vi "Trip Log and Trip Monitor.vi"(8 "error in (no error)":errorcluster, 11 "main ref":T1) -> (0 "error out":errorcluster)   [LabVIEW 2025]
uses:
  controls/LAB-IQ UI Data.ctl
  <vilib>/Utility/error.llb/Trim Whitespace One-Sided.vi
panel:
  in  "millisecond multiple":u32=5
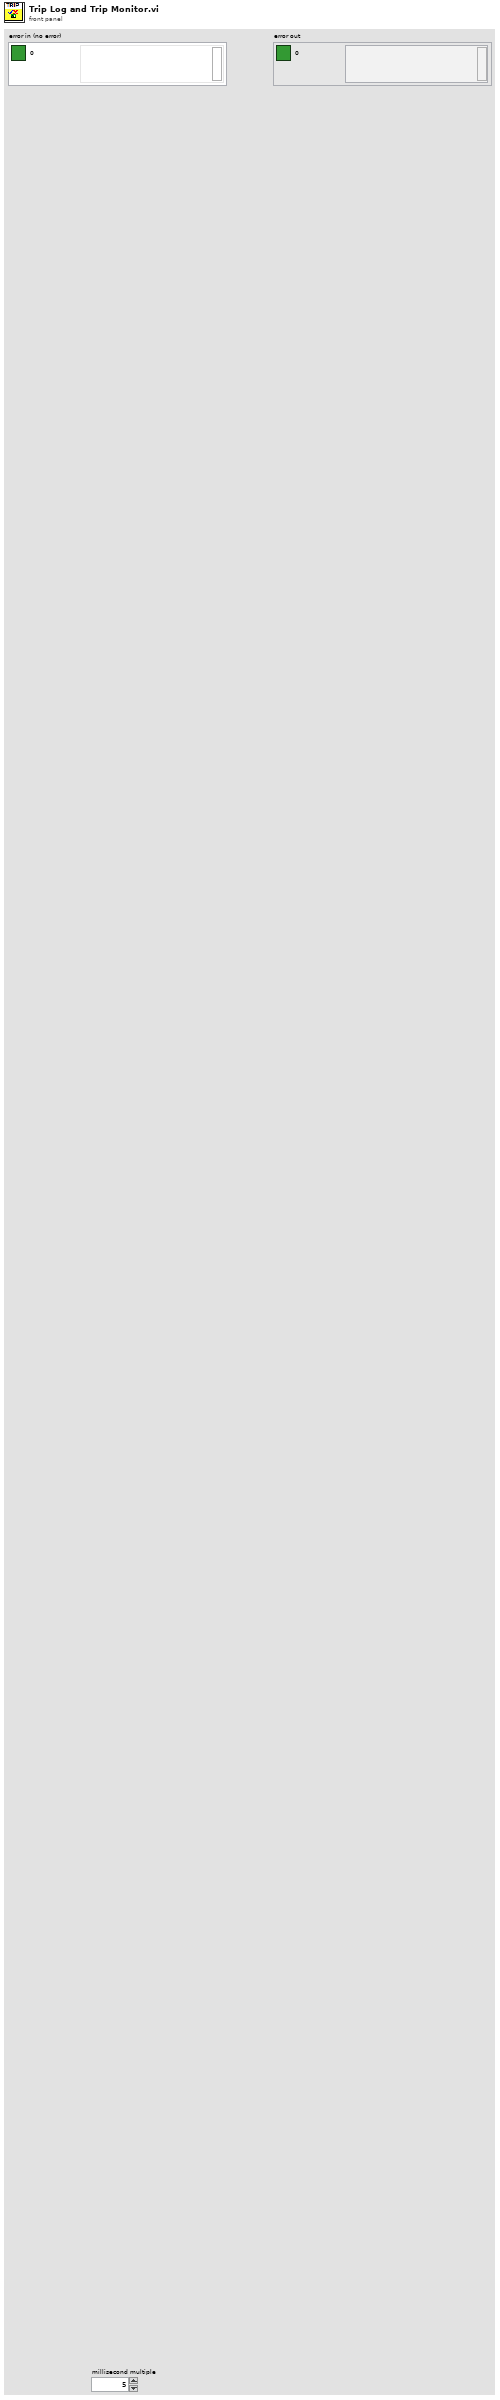
[diagram p1: front panel]
types:
  T1 = typedef "LAB-IQ UI Data.ctl" = cluster{"Main Home Screen":cluster{"GUI":refnum<vi>, "Platform Settings":refnum<vi>, "Configure":refnum<vi>, "Home":refnum<vi>, "EXIT":refnum<vi>, "service 2":refnum<vi>, "MainPage":refnum<vi>, "Analysis":refnum<vi>}, "Platform Settings":cluster{"mm/s  Surge":refnum<vi>, "Update Surge Speed":refnum<vi>, "Drive Error":refnum<vi>, "Disable Axis Jog Soft Limits":refnum<vi>, "mm/s  Sway":refnum<vi>, "Sway and Surge COM Status":refnum<vi>, "Heave COM Status":refnum<vi>, "Enable Platform":refnum<vi>, "Surge Forward Main":refnum<vi>, "Sway Right Main":refnum<vi>, "Sway Left Main":refnum<vi>, "Heave Down Main":refnum<vi>, "Heave Up main":refnum<vi>, "Update Sway Speed":refnum<vi>, "Update Heave Speed":refnum<vi>, "mm/s Heave":refnum<vi>, "mm/sec":refnum<vi>, "mm":refnum<vi>, "Surge Backward Main":refnum<vi>}, "Analysis Screen":cluster{"Analysis Home":refnum<vi>, "Surface Analysis":refnum<vi>, "Imaging":refnum<vi>, "Image Analysis":refnum<vi>, "Post Analysis":refnum<vi>}, "Config Screen":cluster{"Select Load Head":refnum<vi>, "Notes :":refnum<vi>, "FILE":refnum<vi>, "Sample ID :":refnum<vi>, "Operator ID :":refnum<vi>, "Operator Name :":refnum<vi>, "Auto":refnum<vi>}, "Motion Module":cluster{"zNL":refnum<vi>, "NL disp":refnum<vi>, "Rotary Tab":refnum<vi>, "Motion Direction:  3":refnum<vi>, "E.Velocity 2":refnum<vi>, "e.v/ssr 2":refnum<vi>, "Enter Fixed E.Velocity 2":refnum<vi>, "Enter Final SRR 2":refnum<vi>, "Enter initial SRR 2":refnum<vi>, "Enter Fixed SRR 2":refnum<vi>, "Enter the Final E.Velocity (m/s) 2":refnum<vi>, "Enter initial E.Velocity (m/s) 2":refnum<vi>, "Final Speed (RPM) 3":refnum<vi>, "Initial Speed (RPM) 2":refnum<vi>, "Enter the Final Velocity (m/s) 3":refnum<vi>, "Enter initial Velocity (m/s)  3":refnum<vi>, "Ramp Up 2":refnum<vi>, "TEST SELECTION":refnum<vi>, "SPEED SELECTION : ":refnum<vi>, "Angular Oscillation Set":refnum<vi>, "Traction":refnum<vi>, "Step Speed":refnum<vi>, "StepTable For Load-Speed":refnum<vi>, "StepTable For Speed":refnum<vi>, "Surge Forward MM":refnum<vi>, "Surge Backward MM":refnum<vi>, "M3 Image":refnum<vi>, "String 39":refnum<vi>, "Sway Left MM":refnum<vi>, "Sway Right MM":refnum<vi>, "Disable Axis Jog Soft Limits":refnum<vi>, "mm":refnum<vi>, "Heave Down MM":refnum<vi>, "Heave Up MM":refnum<vi>, "Wear Track Diameter (mm)":refnum<vi>, "Set WTD":refnum<vi>, "HomeScratch":refnum<vi>, "HomeRot":refnum<vi>, "PlaceModule":refnum<vi>, "Enter the Angle (Deg)":refnum<vi>, "Enter the Frequency (Hz)":refnum<vi>, "Motion Mode:":refnum<vi>, "LR Sway":refnum<vi>, "Rot Hor":refnum<vi>, "Scratch":refnum<vi>, "LR Cam":refnum<vi>, "MMBack":refnum<vi>, "MMNext":refnum<vi>, "Rot Ver":refnum<vi>, "Rotary Module Selection":refnum<vi>, "calculate rotary":refnum<vi>, "SPEED SELECTION : rotary":refnum<vi>, "Import 2":refnum<vi>, "Save 2":refnum<vi>, "File Path :  2":refnum<vi>, "String 45":refnum<vi>, "StepTable For Speed 3":refnum<vi>, "Enter the Speed(mm/sec)":refnum<vi>, "Enter the Speed(RPM)":refnum<vi>, "Enter Scratch Speed (mm/s):":refnum<vi>, "SwaySpeed Set":refnum<vi>, "Scartch Offset":refnum<vi>, "Motion type:":refnum<vi>, "HomeScratch 2":refnum<vi>, "Enter Scratch length (mm):":refnum<vi>, "Wear Track Diameter":refnum<vi>, "Rotary Speed Exced":refnum<vi>, "Scratch Mode":refnum<vi>, "No of Scratch":refnum<vi>}, "Environmental control":cluster{"Humidity  Status  3":refnum<vi>, "Low Temp  Status  2":refnum<vi>, "TK4 status 2":refnum<vi>, "Stage Temperature":refnum<vi>, "Sample Temperature":refnum<vi>, "Humidity (Amb)":refnum<vi>, "Clear List":refnum<vi>, "Add to list":refnum<vi>, "Wear":refnum<vi>, "Vibration":refnum<vi>, "Humidity (Chamber)":refnum<vi>, "Temperature (Chamber)":refnum<vi>, "ECR ":refnum<vi>, "Temperature (Amb)":refnum<vi>, "Microphone":refnum<vi>, "Acoustic Emission 3":refnum<vi>, "SNext":refnum<vi>, "APBack":refnum<vi>, "Enter the Temperature (°C):":refnum<vi>, "Enter the Stage \nTemperature (°C):":refnum<vi>, "Enter the Humidity (%Rh):":refnum<vi>, "Low Temp":refnum<vi>, "High Temp":refnum<vi>, "Humidity":refnum<vi>, "Sensors Picked":refnum<vi>}, "About Screen":cluster{"Password":refnum<vi>, "Home Service":refnum<vi>, "Advanced Setting":refnum<vi>, "About Tab":refnum<vi>, "ECR Port:":refnum<vi>, "Ramp Port:":refnum<vi>, "Installation/Replacement completed":refnum<vi>, "Loahead":refnum<vi>, "Heave and Surge COM Port:":refnum<vi>, "Sway COM Port:":refnum<vi>, "Temp Modbus:":refnum<vi>, "Humidity Port:":refnum<vi>, "Edit Gain Constants":refnum<vi>, "Save Gain Constants":refnum<vi>}, "Main Screen":cluster{"Main Screen Tab":refnum<vi>, "Angle and Frequency":refnum<vi>, "Stroke (mm)":refnum<vi>, "Angle (Deg)":refnum<vi>, "Main Speed Tab":refnum<vi>, "MTM MOTOR DISPLAY":refnum<vi>, "Disc Speed (m/sec)":refnum<vi>, "Ball Speed (m/sec)":refnum<vi>, "Disc Speed (RPM)":refnum<vi>, "Ball Speed (RPM)":refnum<vi>, "SPEED TAB":refnum<vi>, "Speed (m/sec)":refnum<vi>, "Set Speed (m/sec)":refnum<vi>, "Speed (RPM)":refnum<vi>, "Set Speed":refnum<vi>, "Time Tab":refnum<vi>, "Time ( HH:MM:SS ) 2":refnum<vi>, "Test Duration":refnum<vi>, "Test Duration 4":refnum<vi>, "TEST CYCLE":refnum<vi>, "TOTAL CYCLES":refnum<vi>, "Set Load (N)":refnum<vi>, "Temp Tabs":refnum<vi>, "Heater":refnum<vi>, "TK4 status":refnum<vi>, "ChamberTemp":refnum<vi>, "SetTmp":refnum<vi>, "Controller  Status":refnum<vi>, "ChamberTemp 2":refnum<vi>, "SetTmp 2":refnum<vi>, "Controller  Status 2":refnum<vi>, "ChamberTemp 3":refnum<vi>, "SetTmp 3":refnum<vi>, "Cooling":refnum<vi>, "Load Communication":refnum<vi>, "Ambient \nTemperature":refnum<vi>, "HumCOMStatus":refnum<vi>, "Ambient\n Humidity":refnum<vi>, "Freq (Hz)":refnum<vi>, "Load En":refnum<vi>, "NLt":refnum<vi>, "zNL 2":refnum<vi>, "Humidity On":refnum<vi>, "humidity disp":refnum<vi>, "Set Humidity":refnum<vi>, "NL disp 2":refnum<vi>, "Humidity On 2":refnum<vi>, "humidity disp 2":refnum<vi>, "Set Humidity 2":refnum<vi>, "NL disp 3":refnum<vi>, "AppLoadSeq scratch":refnum<vi>, "Stop Scratch":refnum<vi>, "ClrLog":refnum<vi>, "Trip Log":refnum<vi>, "STOP":refnum<vi>, "Start Test":refnum<vi>, "Test status":refnum<vi>, "AR Led":refnum<vi>, "Data":refnum<vi>, "Health":refnum<vi>, "Sway COM Status":refnum<vi>, "Heave COM Status":refnum<vi>, "Grp Tab":refnum<vi>, "Sub Graph":refnum<vi>, "SD (mm)":refnum<vi>, "Siliding distance Reset Graph":refnum<vi>, "SDGp":refnum<vi>, "Humidity Reset Graph":refnum<vi>, "HumrGp":refnum<vi>, "Acoustic Emission (mV)":refnum<vi>, "Aqucostic Reset Graph":refnum<vi>, "gACQUOS":refnum<vi>, "ECR RESET":refnum<vi>, "ECR":refnum<vi>, "Temperature Reset":refnum<vi>, "Acoustic Emission (mV) 2":refnum<vi>, "Aqucostic Reset Graph 2":refnum<vi>, "gACQUOS 2":refnum<vi>, "ECR RESET 2":refnum<vi>, "ECR 2":refnum<vi>, "Temperature Reset 2":refnum<vi>, "Temperature (deg c)":refnum<vi>, "Speed Reset Graph":refnum<vi>, "Speed Tab":refnum<vi>, "MTM DISC  SPEED":refnum<vi>, "MTM BALL SPEED":refnum<vi>, "speed mm/sec":refnum<vi>, "Hymidity":refnum<vi>, "Humidity Disable trip":refnum<vi>, "CoF Trip  2":refnum<vi>, "Depth Trip":refnum<vi>, "Weart Deapth":refnum<vi>, "Depth Reset Graph":refnum<vi>, "Weart":refnum<vi>, "Depthz":refnum<vi>, "Depth (µm)":refnum<vi>, "WearGp":refnum<vi>, "NL Trip 2":refnum<vi>, "Load pid":refnum<vi>, "Load Disable Trip":refnum<vi>, "Load Reset Graph":refnum<vi>, "NL Display 4":refnum<vi>, "Main Chart 3":refnum<vi>, "BACK":refnum<vi>, "Depth Trip 2":refnum<vi>, "COF TRIP ":refnum<vi>, "Friction Force (N)":refnum<vi>, "FF Reset Graph":refnum<vi>, "FF Disable Trip":refnum<vi>, "FF TRIP":refnum<vi>, "COF Disable Trip":refnum<vi>, "COF Reset Graph":refnum<vi>, "Start Test Temp":refnum<vi>, "zFF":refnum<vi>, "Friction Force (N) Graph":refnum<vi>, "Coefficient of Friction":refnum<vi>, "Scratch Start Test":refnum<vi>, "FF Tab":refnum<vi>, "Cyclic Friction Force (N)":refnum<vi>, "CZ FF":refnum<vi>, "Cyclic Friction Force (N) Graph":refnum<vi>, "Cyclic Coefficient of Friction":refnum<vi>, "Cyclic FF TRIP":refnum<vi>, "Cyclic FF Disable Trip":refnum<vi>, "cyclic COF Disable Trip":refnum<vi>, "cyclic COF TRIP":refnum<vi>, "cyclic COF Reset Graph":refnum<vi>, "Cyclic FF Reset Graph":refnum<vi>, "Test Trip":refnum<vi>, "Multi Scratch Pass":refnum<vi>}, "Loading":cluster{"Indentation":refnum<vi>, "Reference Sample":refnum<vi>, "Load Cell Communication Slide":refnum<vi>, "com 3":refnum<vi>, "com":refnum<vi>, "DecaForce COM Status":refnum<vi>, "Update":refnum<vi>, "Clear 3":refnum<vi>, "seq":refnum<vi>, "Stribeck table":refnum<vi>, "Stribeck Table  For loading":refnum<vi>, "Loading Mode":refnum<vi>, "Enter the Final Load (N)":refnum<vi>, "Enter the CoF Trip":refnum<vi>, "Enter the Friction Force Trip":refnum<vi>, "Enter the Normal load Trip":refnum<vi>, "Enter the Load  (N)":refnum<vi>, "KiloForce":refnum<vi>, "DecaForce ":refnum<vi>, "MicroForce":refnum<vi>, "LHBack":refnum<vi>, "LHNext":refnum<vi>, "Enter the Loading Rate (N/min)":refnum<vi>, "Message":refnum<vi>, "Warning 2":refnum<vi>, "SSP 0.75":refnum<vi>, "SSP 0.5":refnum<vi>, "SSP 0.3":refnum<vi>, "Warning":refnum<vi>, "gui GIF":refnum<vi>, "Communication is established":refnum<vi>, "AppLoad 4":refnum<vi>, "Multipoint":refnum<vi>, "Load Selection":refnum<vi>}, "PID":cluster{"Ramp MulFac":refnum<vi>, "pulses LoadDiffRamp(2..10)":refnum<vi>, "PulseControlRamp(diff<=3N)":refnum<vi>, "SetLoadDeadband(%) Load(0-10N)":refnum<vi>, "PID gains out delay (microForce)":refnum<vi>, "Ramp":refnum<vi>, "Gain 2":refnum<vi>, "pulses LoadDiff(2..10)":refnum<vi>, "pulses LoadDiff(11..50)":refnum<vi>, "PulseControl(diff<=3N)":refnum<vi>, "SetLoadDeadband(%)  2":refnum<vi>, "Dummy Run":refnum<vi>, "Vertical load (N)":refnum<vi>, "AutoTune":refnum<vi>, "Offset 3 ":refnum<vi>, "apply load":refnum<vi>, "Offset  3":refnum<vi>, "apply load 2":refnum<vi>, "Enter ByPass Load":refnum<vi>, "reinit 3":refnum<vi>, "output range delay":refnum<vi>, "PID gains out delay":refnum<vi>, "Bypass Load":refnum<vi>, "pulsesSent":refnum<vi>, "pulses ":refnum<vi>, "actpid":refnum<vi>, "gFF Rot":refnum<vi>, "pulses LoadDiff(21..1000)":refnum<vi>, "Delay":refnum<vi>, "deadband":refnum<vi>}, "Config Parameters":cluster{"Tab Control 3":refnum<vi>, "Tab Control 19":refnum<vi>, "SAMPLES":refnum<vi>, "Re-initilaize":refnum<vi>, "Filter ON/OFF":refnum<vi>, "TracHomeSurgeOffsetCounts 10MM":refnum<vi>, "TracHomeSwayOffsetCounts 10MM":refnum<vi>, "Acoustic Emission:":refnum<vi>, "Apply Filter (FF)":refnum<vi>, "Filter% 2":refnum<vi>, "Apply Filter (Load)":refnum<vi>, "Filter% ":refnum<vi>, "Sway distance (mm)":refnum<vi>, "Surge distance (mm)":refnum<vi>, "DataSavingLoopDelay(ms)":refnum<vi>, "SAVE 2":refnum<vi>, "Enter Distance":refnum<vi>, "Sway Counts:":refnum<vi>, "Distance (mm): 3":refnum<vi>, "Surge Counts:":refnum<vi>, "Distance (mm): 2":refnum<vi>, "Distance (mm):":refnum<vi>, "Heave Counts:":refnum<vi>, "LRMHomeSurgeOffsetCounts":refnum<vi>, "LRMHomeSwayOffsetCounts":refnum<vi>, "TracHomeSurgeOffsetCounts 20MM":refnum<vi>, "TracHomeSwayOffsetCounts 20MM":refnum<vi>, "RotHomeSwayOffsetCounts":refnum<vi>, "RotHomeSurgeOffsetCounts":refnum<vi>, "Heave distance":refnum<vi>, "Zmm":refnum<vi>, "Heave Pulses/mm":refnum<vi>, "Surge Pulses/mm":refnum<vi>, "Sway Pulses/mm":refnum<vi>, "Heave Pitch":refnum<vi>, "Surge Pitch":refnum<vi>, "Sway Pitch":refnum<vi>, "Heave PPR":refnum<vi>, "Surge PPR":refnum<vi>, "Sway PPR":refnum<vi>, "Tab Control 5":refnum<vi>, "Tab Control 14":refnum<vi>, "Tab Control 26":refnum<vi>, "AE":refnum<vi>, "Heave Loop Delay":refnum<vi>, "Heave PID Speed":refnum<vi>, "Surge Jog Speed":refnum<vi>, "Heave Jog Speed":refnum<vi>, "Sway Loop Delay":refnum<vi>, "Sway PID Speed":refnum<vi>, "Sway Jog Speed":refnum<vi>}, "Loading Com Port":cluster{"ClearAll":refnum<vi>, "Mz(Nm)":refnum<vi>, "My(Nm)":refnum<vi>, "Mx(Nm)":refnum<vi>, "Save Dwell":refnum<vi>, "Mx ":refnum<vi>, "My ":refnum<vi>, "Mz":refnum<vi>, "Fx(N)":refnum<vi>, "Fy(N)":refnum<vi>, "Fz(N)":refnum<vi>, "ZeroAll":refnum<vi>, "Acq Delay (ms)":refnum<vi>, "Burst Delay (ms)":refnum<vi>, "model":refnum<vi>, "SN":refnum<vi>, "FFx(N)":refnum<vi>, "Sensor IP":refnum<vi>, "Port":refnum<vi>, "FFy(N)":refnum<vi>, "Load(N)":refnum<vi>, "delete Handle":refnum<vi>, "Create Handle":refnum<vi>, "ft_data":refnum<vi>, "ft_range":refnum<vi>, "ft_data 2":refnum<vi>, "stop 6":refnum<vi>, "running_flag":refnum<vi>, "ft_udp_handle":refnum<vi>, "get-data-return":refnum<vi>, "get-range-return":refnum<vi>, "zero-return":refnum<vi>, "filter-return":refnum<vi>, "initial-return":refnum<vi>, "deleteHandle-result":refnum<vi>, "Load Cell Temp":refnum<vi>}, "Heave AND Surge":cluster{"SURGE POSE":refnum<vi>, "error out Read":refnum<vi>, "HEAVE POSE":refnum<vi>, "State":refnum<vi>, "Homed":refnum<vi>, "Sequence ID":refnum<vi>, "error out Write":refnum<vi>, "faultCode":refnum<vi>, "Ack ID":refnum<vi>, "SPEED":refnum<vi>, "Distance":refnum<vi>, "Mode Command":refnum<vi>, "Heave and Surge Read":refnum<vi>, "Read Heave Temp":refnum<vi>, "Spare 15":refnum<vi>, "Spare 14":refnum<vi>, "Spare 13":refnum<vi>, "Spare 12":refnum<vi>, "Spare 11":refnum<vi>, "Spare 10":refnum<vi>, "Spare 9":refnum<vi>, "Spare 8":refnum<vi>, "Spare 7":refnum<vi>, "Spare 6":refnum<vi>, "Spare 5":refnum<vi>, "Spare 4":refnum<vi>, "Spare 2":refnum<vi>, "Spare 1":refnum<vi>, "Node Id":refnum<vi>, "Spare 3":refnum<vi>, "SPARE 4":refnum<vi>, "SPARE 3":refnum<vi>, "SPARE 2":refnum<vi>, "SPARE 1":refnum<vi>, "fwMajor":refnum<vi>, "fwMinor":refnum<vi>, "Manual Write":refnum<vi>, "Heave and Surge Write":refnum<vi>}, "New PID LOGIC":cluster{"Fine Tune Zone":refnum<vi>, "PID SDelay":refnum<vi>, "Max_pos_limit":refnum<vi>, "Min_pos_limit":refnum<vi>, "i_limit":refnum<vi>, "pct_scale":refnum<vi>, "Deadband":refnum<vi>, "Kd":refnum<vi>, "Ki":refnum<vi>, "Kp":refnum<vi>, "Current Position":refnum<vi>, "Set Load":refnum<vi>, "Current Load":refnum<vi>, "Pulse delta":refnum<vi>, "Init Step":refnum<vi>, "Max Step Linit":refnum<vi>}, "SWAY ":cluster{"fwMajor":refnum<vi>, "Homed":refnum<vi>, "Rotary POSE":refnum<vi>, "State":refnum<vi>, "SWAY POSE":refnum<vi>, "Ack ID":refnum<vi>, "faultCode":refnum<vi>, "Node Id":refnum<vi>, "fwMinor":refnum<vi>, "Spare 6":refnum<vi>, "Spare 5":refnum<vi>, "Spare 4":refnum<vi>, "Spare 3":refnum<vi>, "Spare 2":refnum<vi>, "Spare 1":refnum<vi>, "Spare 7":refnum<vi>, "SPARE  5":refnum<vi>, "error out Write  SWAY ":refnum<vi>, "error out Read SWAY ":refnum<vi>, "Manual Write SWAY ":refnum<vi>, "SWAY WRITE":refnum<vi>, "SPARE  4":refnum<vi>, "SPARE  3":refnum<vi>, "SPARE 2":refnum<vi>, "SPARE 1":refnum<vi>, "Spare 15":refnum<vi>, "Spare 14":refnum<vi>, "Spare 13":refnum<vi>, "Spare 12":refnum<vi>, "Spare 11":refnum<vi>, "Spare 9":refnum<vi>, "Spare 8":refnum<vi>, "SPEED":refnum<vi>, "Distance":refnum<vi>, "Mode Command":refnum<vi>, "Sequence ID":refnum<vi>, "SWAY READ":refnum<vi>, "Spare 10":refnum<vi>, "Read SWAY Temp":refnum<vi>}, "Analysis Screen":cluster{"Analysis Home":refnum<vi>, "Refresh 2":refnum<vi>, "MEAN 4":refnum<vi>, "SD 4":refnum<vi>, "VARIANCE 4":refnum<vi>, "MEAN  3":refnum<vi>, "SD  3":refnum<vi>, "VARIANCE  3":refnum<vi>, "MEAN 2":refnum<vi>, "SD  2":refnum<vi>, "VARIANCE 2":refnum<vi>, "MEAN":refnum<vi>, "SD":refnum<vi>, "VARIANCE":refnum<vi>, "File 4 Discription":refnum<vi>, "OPEN 4":refnum<vi>, "File Name 4":refnum<vi>, "OPEN 3":refnum<vi>, "File 3 Discription":refnum<vi>, "File Name 3":refnum<vi>, "Y-AXIS":refnum<vi>, "X-AXIS":refnum<vi>, "XY Graph":refnum<vi>, "File Name 2":refnum<vi>, "File Name 1":refnum<vi>, "OPEN 2":refnum<vi>, "OPEN 1":refnum<vi>, "File 1 Discription ":refnum<vi>, "File 2 Discription":refnum<vi>}}
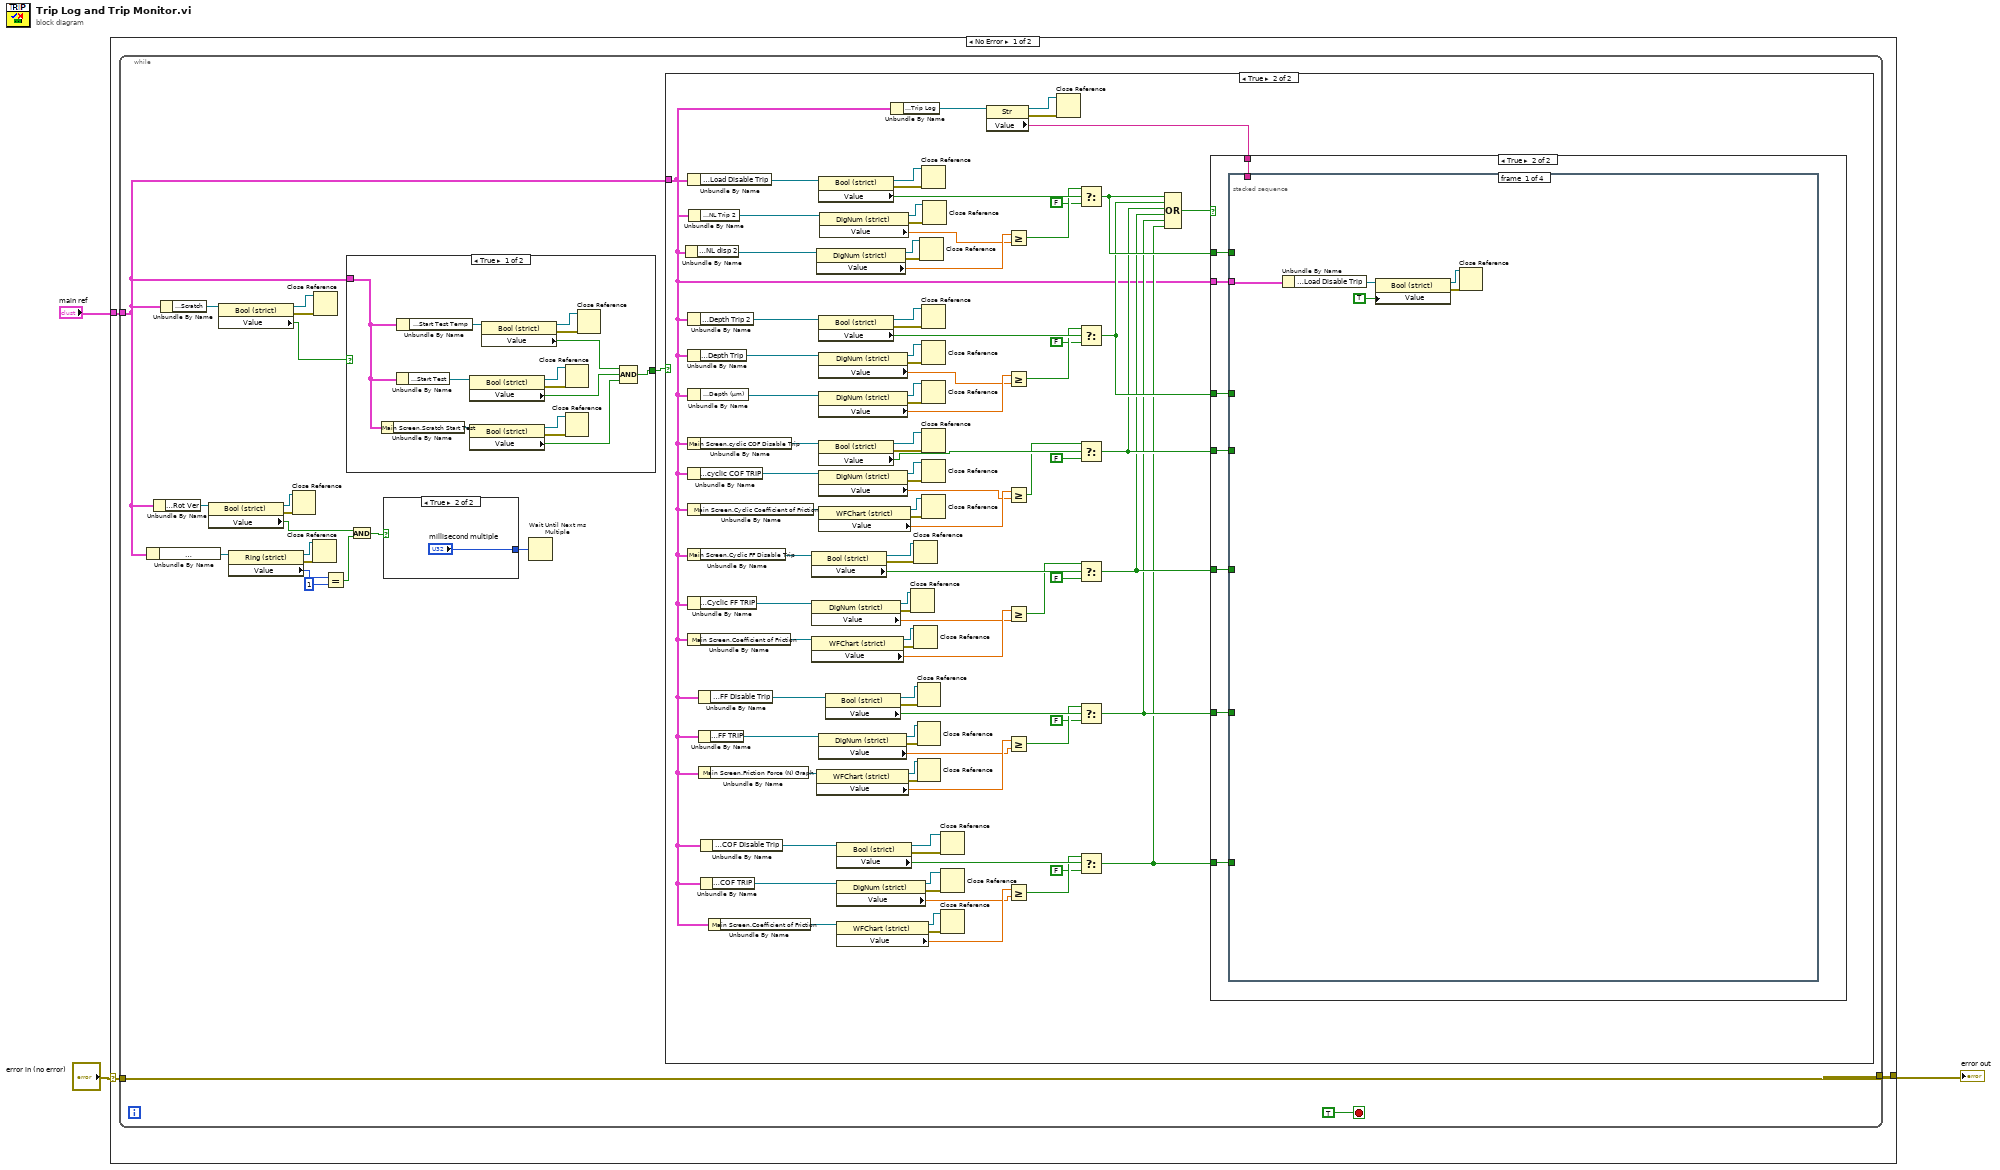
[diagram p0: block diagram]
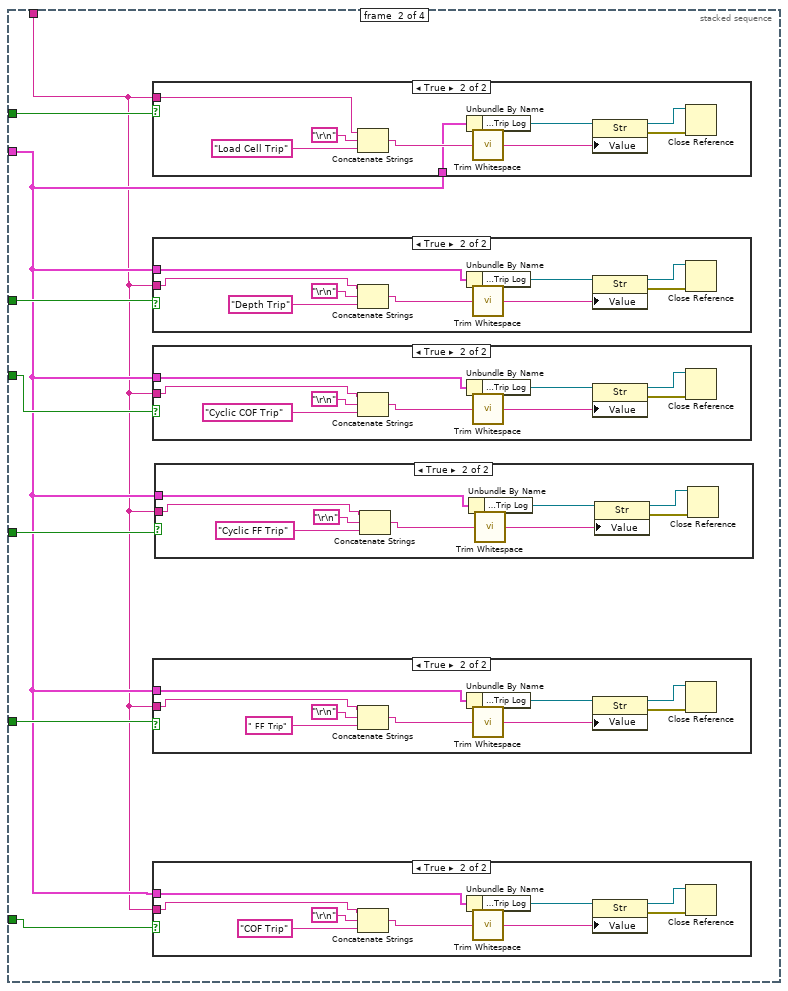
[diagram p4: hidden frame]
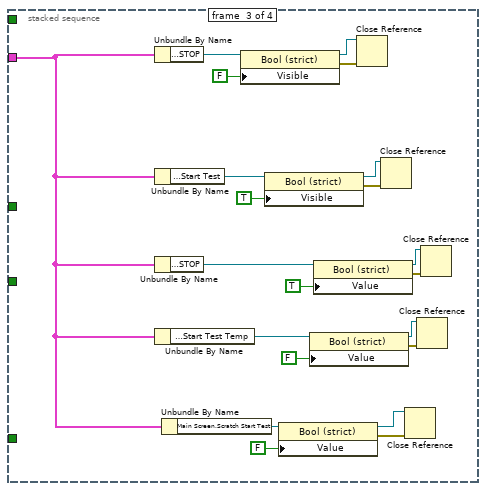
[diagram p11: hidden frame]
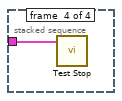
[diagram p12: hidden frame]
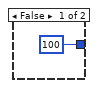
[diagram p13: hidden frame]
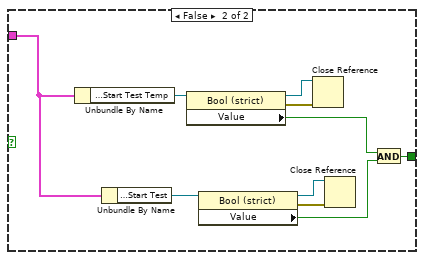
[diagram p14: hidden frame]
diagram:
  n1 = case shown="No Error" "error in (no error)" {
    selector: "error in (no error)" -> [w6 _]
    tunnel: [w5 _] -> w2
    tunnel: "main ref" -> [w4 _]
    frame No Error {
      n2 = while {
        tunnel: [w9] -> w5
        tunnel: w6 -> [w9]
        tunnel: w4 -> [w7]
        stop <- TRUE stop-if-true
        n3 = Unbundle By Name(w7) -> ("Motion Module.Motion Mode:"=w16:refnum<vi>)
        n4 = Unbundle By Name(w7) -> ("Motion Module.Rot Ver"=w21:refnum<vi>)
        n5 = Unbundle By Name(w7) -> ("Motion Module.Scratch"=w25:refnum<vi>)
        n6 = property class="Bool (strict)"(reference=w21) -> (reference out=w19:refnum<vi>, error out=w20:errorcluster, "Value"=w13:bool)  [unwired: 1 in]
        n7 = property class="Bool (strict)"(reference=w25) -> (reference out=w26:refnum<vi>, error out=w24:errorcluster, "Value"=w23:bool)  [unwired: 1 in]
        n8 = property class="Ring (strict)"(reference=w16) -> (reference out=w18:refnum<vi>, error out=w17:errorcluster, "Value"=w15:u16)  [unwired: 1 in]
        n9 = Close Reference(reference=w19, error in (no error)=w20) -> ()  [unwired: 1 out]
        n10 = Close Reference(reference=w18, error in (no error)=w17) -> ()  [unwired: 1 out]
        n11 = Close Reference(reference=w26, error in (no error)=w24) -> ()  [unwired: 1 out]
        n12 = Equal?(x=w15, y=u16 1) -> (x = y?=w12:bool)
        n13 = case shown="True" w23 {
          tunnel: w7 -> [w223 w239]
          tunnel: [w227 w237] -> w8
          frame True {
            n14 = Unbundle By Name(w223) -> ("Main Screen.Scratch Start Test"=w225:refnum<vi>)
            n15 = Unbundle By Name(w223) -> ("Main Screen.Start Test"=w231:refnum<vi>)
            n16 = Unbundle By Name(w223) -> ("Main Screen.Start Test Temp"=w234:refnum<vi>)
            n17 = property class="Bool (strict)"(reference=w231) -> (reference out=w230:refnum<vi>, error out=w232:errorcluster, "Value"=w228:bool)  [unwired: 1 in]
            n18 = property class="Bool (strict)"(reference=w225) -> (reference out=w226:refnum<vi>, error out=w224:errorcluster, "Value"=w222:bool)  [unwired: 1 in]
            n19 = property class="Bool (strict)"(reference=w234) -> (reference out=w235:refnum<vi>, error out=w233:errorcluster, "Value"=w229:bool)  [unwired: 1 in]
            n20 = Close Reference(reference=w230, error in (no error)=w232) -> ()  [unwired: 1 out]
            n21 = Close Reference(reference=w226, error in (no error)=w224) -> ()  [unwired: 1 out]
            n22 = Close Reference(reference=w235, error in (no error)=w233) -> ()  [unwired: 1 out]
            n23 = Compound Arithmetic op=AND(w229, w228, w222) -> (w227:bool)
          }
          frame False {
            n24 = Unbundle By Name(w239) -> ("Main Screen.Start Test Temp"=w244:refnum<vi>)
            n25 = Unbundle By Name(w239) -> ("Main Screen.Start Test"=w241:refnum<vi>)
            n26 = property class="Bool (strict)"(reference=w244) -> (reference out=w245:refnum<vi>, error out=w243:errorcluster, "Value"=w238:bool)  [unwired: 1 in]
            n27 = property class="Bool (strict)"(reference=w241) -> (reference out=w240:refnum<vi>, error out=w242:errorcluster, "Value"=w236:bool)  [unwired: 1 in]
            n28 = Close Reference(reference=w245, error in (no error)=w243) -> ()  [unwired: 1 out]
            n29 = Close Reference(reference=w240, error in (no error)=w242) -> ()  [unwired: 1 out]
            n30 = And(x=w238, y=w236) -> (x .and. y?=w237:bool)
          }
        }
        n31 = And(x=w13, y=w12) -> (x .and. y?=w11:bool)
        n32 = case shown="True" w11 {
          tunnel: [u32 100 ("millisecond multiple") "millisecond multiple"] -> w22
          frame False {
          }
          frame True {
          }
        }
        n33 = Wait Until Next ms Multiple(millisecond multiple=w22) -> ()  [unwired: 1 out]
        n34 = case shown="True" w8 {
          tunnel: w7 -> [_ w28]
          frame False {
          }
          frame True {
            n35 = Unbundle By Name(w28) -> ("Main Screen.NL disp 2"=w122:refnum<vi>)
            n36 = Unbundle By Name(w28) -> ("Main Screen.Load Disable Trip"=w99:refnum<vi>)
            n37 = Unbundle By Name(w28) -> ("Main Screen.Depth Trip 2"=w94:refnum<vi>)
            n38 = Unbundle By Name(w28) -> ("Main Screen.Depth Trip"=w97:refnum<vi>)
            n39 = Unbundle By Name(w28) -> ("Main Screen.Depth (µm)"=w119:refnum<vi>)
            n40 = Unbundle By Name(w28) -> ("Main Screen.cyclic COF Disable Trip"=w91:refnum<vi>)
            n41 = Unbundle By Name(w28) -> ("Main Screen.cyclic COF TRIP"=w88:refnum<vi>)
            n42 = Unbundle By Name(w28) -> ("Main Screen.Cyclic Coefficient of Friction"=w116:refnum<vi>)
            n43 = Unbundle By Name(w28) -> ("Main Screen.Cyclic FF Disable Trip"=w82:refnum<vi>)
            n44 = Unbundle By Name(w28) -> ("Main Screen.Cyclic FF TRIP"=w85:refnum<vi>)
            n45 = Unbundle By Name(w28) -> ("Main Screen.Coefficient of Friction"=w113:refnum<vi>)
            n46 = Unbundle By Name(w28) -> ("Main Screen.NL Trip 2"=w102:refnum<vi>)
            n47 = Unbundle By Name(w28) -> ("Main Screen.FF Disable Trip"=w109:refnum<vi>)
            n48 = Unbundle By Name(w28) -> ("Main Screen.FF TRIP"=w80:refnum<vi>)
            n49 = Unbundle By Name(w28) -> ("Main Screen.Friction Force (N) Graph"=w75:refnum<vi>)
            n50 = Unbundle By Name(w28) -> ("Main Screen.COF TRIP"=w71:refnum<vi>)
            n51 = Unbundle By Name(w28) -> ("Main Screen.COF Disable Trip"=w72:refnum<vi>)
            n52 = Unbundle By Name(w28) -> ("Main Screen.Coefficient of Friction"=w108:refnum<vi>)
            n53 = property class="Bool (strict)"(reference=w82) -> (reference out=w83:refnum<vi>, error out=w81:errorcluster, "Value"=w65:bool)  [unwired: 1 in]
            n54 = property class="DigNum (strict)"(reference=w85) -> (reference out=w84:refnum<vi>, error out=w86:errorcluster, "Value"=w52:dbl)  [unwired: 1 in]
            n55 = property class="WFChart (strict)"(reference=w113) -> (reference out=w114:refnum<vi>, error out=w112:errorcluster, "Value"=w53:dbl)  [unwired: 1 in]
            n56 = property class="DigNum (strict)"(reference=w122) -> (reference out=w105:refnum<vi>, error out=w121:errorcluster, "Value"=w62:dbl)  [unwired: 1 in]
            n57 = property class="WFChart (strict)"(reference=w75) -> (reference out=w76:refnum<vi>, error out=w77:errorcluster, "Value"=w50:dbl)  [unwired: 1 in]
            n58 = property class="DigNum (strict)"(reference=w80) -> (reference out=w79:refnum<vi>, error out=w78:errorcluster, "Value"=w49:dbl)  [unwired: 1 in]
            n59 = property class="Bool (strict)"(reference=w99) -> (reference out=w101:refnum<vi>, error out=w100:errorcluster, "Value"=w68:bool)  [unwired: 1 in]
            n60 = property class="Bool (strict)"(reference=w94) -> (reference out=w95:refnum<vi>, error out=w93:errorcluster, "Value"=w67:bool)  [unwired: 1 in]
            n61 = property class="DigNum (strict)"(reference=w97) -> (reference out=w96:refnum<vi>, error out=w98:errorcluster, "Value"=w58:dbl)  [unwired: 1 in]
            n62 = property class="DigNum (strict)"(reference=w119) -> (reference out=w120:refnum<vi>, error out=w118:errorcluster, "Value"=w59:dbl)  [unwired: 1 in]
            n63 = property class="Bool (strict)"(reference=w91) -> (reference out=w92:refnum<vi>, error out=w90:errorcluster, "Value"=w66:bool)  [unwired: 1 in]
            n64 = property class="DigNum (strict)"(reference=w88) -> (reference out=w87:refnum<vi>, error out=w89:errorcluster, "Value"=w55:dbl)  [unwired: 1 in]
            n65 = property class="WFChart (strict)"(reference=w116) -> (reference out=w115:refnum<vi>, error out=w117:errorcluster, "Value"=w56:dbl)  [unwired: 1 in]
            n66 = property class="DigNum (strict)"(reference=w102) -> (reference out=w104:refnum<vi>, error out=w103:errorcluster, "Value"=w61:dbl)  [unwired: 1 in]
            n67 = property class="Bool (strict)"(reference=w109) -> (reference out=w110:refnum<vi>, error out=w111:errorcluster, "Value"=w64:bool)  [unwired: 1 in]
            n68 = property class="Bool (strict)"(reference=w72) -> (reference out=w74:refnum<vi>, error out=w73:errorcluster, "Value"=w63:bool)  [unwired: 1 in]
            n69 = property class="DigNum (strict)"(reference=w71) -> (reference out=w69:refnum<vi>, error out=w70:errorcluster, "Value"=w46:dbl)  [unwired: 1 in]
            n70 = property class="WFChart (strict)"(reference=w108) -> (reference out=w106:refnum<vi>, error out=w107:errorcluster, "Value"=w47:dbl)  [unwired: 1 in]
            n71 = Unbundle By Name(w28) -> ("Main Screen.Trip Log"=w29:refnum<vi>)
            n72 = Close Reference(reference=w84, error in (no error)=w86) -> ()  [unwired: 1 out]
            n73 = Close Reference(reference=w83, error in (no error)=w81) -> ()  [unwired: 1 out]
            n74 = Close Reference(reference=w114, error in (no error)=w112) -> ()  [unwired: 1 out]
            n75 = Close Reference(reference=w110, error in (no error)=w111) -> ()  [unwired: 1 out]
            n76 = Close Reference(reference=w79, error in (no error)=w78) -> ()  [unwired: 1 out]
            n77 = Close Reference(reference=w76, error in (no error)=w77) -> ()  [unwired: 1 out]
            n78 = Close Reference(reference=w105, error in (no error)=w121) -> ()  [unwired: 1 out]
            n79 = Close Reference(reference=w101, error in (no error)=w100) -> ()  [unwired: 1 out]
            n80 = Close Reference(reference=w95, error in (no error)=w93) -> ()  [unwired: 1 out]
            n81 = Close Reference(reference=w96, error in (no error)=w98) -> ()  [unwired: 1 out]
            n82 = Close Reference(reference=w120, error in (no error)=w118) -> ()  [unwired: 1 out]
            n83 = Close Reference(reference=w92, error in (no error)=w90) -> ()  [unwired: 1 out]
            n84 = Close Reference(reference=w87, error in (no error)=w89) -> ()  [unwired: 1 out]
            n85 = Close Reference(reference=w115, error in (no error)=w117) -> ()  [unwired: 1 out]
            n86 = Close Reference(reference=w104, error in (no error)=w103) -> ()  [unwired: 1 out]
            n87 = Close Reference(reference=w74, error in (no error)=w73) -> ()  [unwired: 1 out]
            n88 = Close Reference(reference=w69, error in (no error)=w70) -> ()  [unwired: 1 out]
            n89 = Close Reference(reference=w106, error in (no error)=w107) -> ()  [unwired: 1 out]
            n90 = property class="Str"(reference=w29) -> (reference out=w30:refnum<vi>, error out=w31:errorcluster, "Value"=w27:string)  [unwired: 1 in]
            n91 = Greater Or Equal?(x=w62, y=w61) -> (x >= y?=w60:bool)
            n92 = Greater Or Equal?(x=w59, y=w58) -> (x >= y?=w57:bool)
            n93 = Greater Or Equal?(x=w56, y=w55) -> (x >= y?=w54:bool)
            n94 = Greater Or Equal?(x=w53, y=w52) -> (x >= y?=w51:bool)
            n95 = Greater Or Equal?(x=w50, y=w49) -> (x >= y?=w48:bool)
            n96 = Greater Or Equal?(x=w47, y=w46) -> (x >= y?=w45:bool)
            n97 = Close Reference(reference=w30, error in (no error)=w31) -> ()  [unwired: 1 out]
            n98 = Select(t=w60, s=w68, f=FALSE) -> (s? t:f=w37:bool)
            n99 = Select(t=w57, s=w67, f=FALSE) -> (s? t:f=w36:bool)
            n100 = Select(t=w54, s=w66, f=FALSE) -> (s? t:f=w35:bool)
            n101 = Select(t=w51, s=w65, f=FALSE) -> (s? t:f=w34:bool)
            n102 = Select(t=w48, s=w64, f=FALSE) -> (s? t:f=w33:bool)
            n103 = Select(t=w45, s=w63, f=FALSE) -> (s? t:f=w32:bool)
            n104 = Compound Arithmetic op=OR(w37, w36, w35, w34, w33, w32) -> (w38:bool)
            n105 = case shown="True" w38 {
              tunnel: w28 -> [_ w130]
              tunnel: w37 -> [_ w129]
              tunnel: w36 -> [_ w128]
              tunnel: w35 -> [_ w127]
              tunnel: w34 -> [_ w126]
              tunnel: w33 -> [_ w125]
              tunnel: w32 -> [_ w124]
              tunnel: w27 -> [_ w123]
              frame False {
              }
              frame True {
                n106 = stacked-sequence {
                  tunnel: w130 -> [w132 w137 w198 w219]
                  tunnel: w129 -> [_ w143 _ _]
                  tunnel: w128 -> [_ w142 _ _]
                  tunnel: w127 -> [_ w141 _ _]
                  tunnel: w126 -> [_ w140 _ _]
                  tunnel: w125 -> [_ w139 _ _]
                  tunnel: w124 -> [_ w138 _ _]
                  tunnel: w123 -> [_ w136 _ _]
                  frame #0 {
                    n107 = Unbundle By Name(w132) -> ("Main Screen.Load Disable Trip"=w133:refnum<vi>)
                    n108 = property class="Bool (strict)"(reference=w133, "Value"=TRUE) -> (reference out=w135:refnum<vi>, error out=w134:errorcluster)  [unwired: 1 in]
                    n109 = Close Reference(reference=w135, error in (no error)=w134) -> ()  [unwired: 1 out]
                  }
                  frame #1 {
                    n110 = case shown="True" w143 {
                      tunnel: w137 -> [_ w191]
                      tunnel: w136 -> [_ w189]
                      frame False {
                      }
                      frame True {
                        n111 = Concatenate Strings(w189, "\r\n", "Load Cell Trip" ("string")) -> (w193:string)
                        n112 = Unbundle By Name(w191) -> ("Main Screen.Trip Log"=w190:refnum<vi>)
                        n113 = call <vilib>:"Trim Whitespace.vi"("string"=w193) -> ("trimmed string"=w192:string)  [unwired: 1 in]
                        n114 = property class="Str"(reference=w190, "Value"=w192) -> (reference out=w194:refnum<vi>, error out=w195:errorcluster)  [unwired: 1 in]
                        n115 = Close Reference(reference=w194, error in (no error)=w195) -> ()  [unwired: 1 out]
                      }
                    }
                    n116 = case shown="True" w142 {
                      tunnel: w137 -> [_ w181]
                      tunnel: w136 -> [_ w180]
                      frame False {
                      }
                      frame True {
                        n117 = Concatenate Strings(w180, "\r\n", "Depth Trip" ("string")) -> (w184:string)
                        n118 = Unbundle By Name(w181) -> ("Main Screen.Trip Log"=w182:refnum<vi>)
                        n119 = call <vilib>:"Trim Whitespace.vi"("string"=w184) -> ("trimmed string"=w183:string)  [unwired: 1 in]
                        n120 = property class="Str"(reference=w182, "Value"=w183) -> (reference out=w185:refnum<vi>, error out=w186:errorcluster)  [unwired: 1 in]
                        n121 = Close Reference(reference=w185, error in (no error)=w186) -> ()  [unwired: 1 out]
                      }
                    }
                    n122 = case shown="True" w141 {
                      tunnel: w137 -> [_ w172]
                      tunnel: w136 -> [_ w171]
                      frame False {
                      }
                      frame True {
                        n123 = Concatenate Strings(w171, "\r\n", "Cyclic COF Trip" ("string")) -> (w175:string)
                        n124 = Unbundle By Name(w172) -> ("Main Screen.Trip Log"=w173:refnum<vi>)
                        n125 = call <vilib>:"Trim Whitespace.vi"("string"=w175) -> ("trimmed string"=w174:string)  [unwired: 1 in]
                        n126 = property class="Str"(reference=w173, "Value"=w174) -> (reference out=w176:refnum<vi>, error out=w177:errorcluster)  [unwired: 1 in]
                        n127 = Close Reference(reference=w176, error in (no error)=w177) -> ()  [unwired: 1 out]
                      }
                    }
                    n128 = case shown="True" w139 {
                      tunnel: w137 -> [_ w154]
                      tunnel: w136 -> [_ w153]
                      frame False {
                      }
                      frame True {
                        n129 = Concatenate Strings(w153, "\r\n", " FF Trip" ("string")) -> (w157:string)
                        n130 = Unbundle By Name(w154) -> ("Main Screen.Trip Log"=w155:refnum<vi>)
                        n131 = call <vilib>:"Trim Whitespace.vi"("string"=w157) -> ("trimmed string"=w156:string)  [unwired: 1 in]
                        n132 = property class="Str"(reference=w155, "Value"=w156) -> (reference out=w158:refnum<vi>, error out=w159:errorcluster)  [unwired: 1 in]
                        n133 = Close Reference(reference=w158, error in (no error)=w159) -> ()  [unwired: 1 out]
                      }
                    }
                    n134 = case shown="True" w138 {
                      tunnel: w137 -> [_ w145]
                      tunnel: w136 -> [_ w144]
                      frame False {
                      }
                      frame True {
                        n135 = Concatenate Strings(w144, "\r\n", "COF Trip" ("string")) -> (w148:string)
                        n136 = Unbundle By Name(w145) -> ("Main Screen.Trip Log"=w146:refnum<vi>)
                        n137 = call <vilib>:"Trim Whitespace.vi"("string"=w148) -> ("trimmed string"=w147:string)  [unwired: 1 in]
                        n138 = property class="Str"(reference=w146, "Value"=w147) -> (reference out=w149:refnum<vi>, error out=w150:errorcluster)  [unwired: 1 in]
                        n139 = Close Reference(reference=w149, error in (no error)=w150) -> ()  [unwired: 1 out]
                      }
                    }
                    n140 = case shown="True" w140 {
                      tunnel: w137 -> [_ w163]
                      tunnel: w136 -> [_ w162]
                      frame False {
                      }
                      frame True {
                        n141 = Concatenate Strings(w162, "\r\n", "Cyclic FF Trip" ("string")) -> (w166:string)
                        n142 = Unbundle By Name(w163) -> ("Main Screen.Trip Log"=w164:refnum<vi>)
                        n143 = call <vilib>:"Trim Whitespace.vi"("string"=w166) -> ("trimmed string"=w165:string)  [unwired: 1 in]
                        n144 = property class="Str"(reference=w164, "Value"=w165) -> (reference out=w167:refnum<vi>, error out=w168:errorcluster)  [unwired: 1 in]
                        n145 = Close Reference(reference=w167, error in (no error)=w168) -> ()  [unwired: 1 out]
                      }
                    }
                  }
                  frame #2 {
                    n146 = Unbundle By Name(w198) -> ("Main Screen.STOP"=w213:refnum<vi>)
                    n147 = Unbundle By Name(w198) -> ("Main Screen.Start Test"=w216:refnum<vi>)
                    n148 = Unbundle By Name(w198) -> ("Main Screen.STOP"=w207:refnum<vi>)
                    n149 = Unbundle By Name(w198) -> ("Main Screen.Start Test Temp"=w206:refnum<vi>)
                    n150 = Unbundle By Name(w198) -> ("Main Screen.Scratch Start Test"=w201:refnum<vi>)
                    n151 = property class="Bool (strict)"(reference=w213, "Visible"=FALSE) -> (reference out=w203:refnum<vi>, error out=w212:errorcluster)  [unwired: 1 in]
                    n152 = property class="Bool (strict)"(reference=w216, "Visible"=TRUE) -> (reference out=w218:refnum<vi>, error out=w217:errorcluster)  [unwired: 1 in]
                    n153 = property class="Bool (strict)"(reference=w201, "Value"=FALSE) -> (reference out=w202:refnum<vi>, error out=w200:errorcluster)  [unwired: 1 in]
                    n154 = property class="Bool (strict)"(reference=w206, "Value"=FALSE) -> (reference out=w204:refnum<vi>, error out=w205:errorcluster)  [unwired: 1 in]
                    n155 = property class="Bool (strict)"(reference=w207, "Value"=TRUE) -> (reference out=w209:refnum<vi>, error out=w208:errorcluster)  [unwired: 1 in]
                    n156 = Close Reference(reference=w203, error in (no error)=w212) -> ()  [unwired: 1 out]
                    n157 = Close Reference(reference=w218, error in (no error)=w217) -> ()  [unwired: 1 out]
                    n158 = Close Reference(reference=w202, error in (no error)=w200) -> ()  [unwired: 1 out]
                    n159 = Close Reference(reference=w204, error in (no error)=w205) -> ()  [unwired: 1 out]
                    n160 = Close Reference(reference=w209, error in (no error)=w208) -> ()  [unwired: 1 out]
                  }
                  frame #3 {
                    n161 = call "Test Stop.vi"("Data Cluster"=w219) -> ()  [unwired: 10 in, 1 out]
                  }
                }
              }
            }
          }
        }
      }
    }
    frame Error {
    }
  }
  "error out" <- w2
